vi "master_python_v1.0.vi"() -> ()   [LabVIEW 2026]
uses:
  <vilib>/Utility/error.llb/DialogType.ctl
  <vilib>/DAQmx/write.llb/DAQmx Write (Analog 2D DBL NChan NSamp).vi
  <vilib>/DAQmx/read.llb/DAQmx Read (Analog 1D Wfm NChan NSamp Duration).vi
  <vilib>/DAQmx/read.llb/DAQmx Read (Analog 1D Wfm NChan NSamp).vi
  <vilib>/DAQmx/miscellaneous.llb/DAQmx Fill In Error Info.vi
  <vilib>/Utility/inputDevices.llb/keyboardAcquire.vi
  Nanostage/Madlib.dll
panel:
  out "PID output":dbl format="%.2f"
  out "Setpoint":dbl
  in  "PID gains":T1={"proportional gain (Kc)"=0.5, "integral time (Ti, min)"=0.0, "derivative time (Td, min)"=0.0} {"derivative time (Td, min)" min=-1e-18 max=1000000000000000.0 step=1e-05 format="%.3f"; "integral time (Ti, min)" min=-1e-18 step=1e-05 format="%.6f"; "proportional gain (Kc)" min=-1e-18 step=1e-05 format="%.5f"}
  in  "output range":cluster{"output high":dbl, "output low":dbl}={"output high"=0.1, "output low"=-0.1} {"output low" format="%.2f"; "output high" format="%.2f"}
  in  "dt (s)":dbl=-1.0 format="%.3f"
  out "QPD":dbl
  out "Pos 0":dbl
  in  "Comment":string
  out "loop iteration":i32
  out "x start":dbl
  out "y start":dbl
  out "z start":dbl
  out "start iteration":dbl
  out "data":waveform(dbl)[](array[waveform])
  out "Numeric 2":i32
  out "Numeric":i32
  out "stop Ind":bool
  in  "Tab Control":enum32{"Main Control", "Calibration"}(tab)
  in  "Apply Force":bool
  out "Waveform Chart 6":waveform(dbl)(graph)
  out "Waveform Chart 5":waveform(dbl)(graph)
  in  "stop":bool
  in  "Record Data":bool
  in  "New File?":bool caption="new_file"
  out "QPD Position":cluster{"Array":dbl[], "Array":dbl[]}(graph)
  out "MT channels":waveform(dbl)[](graph)
  out "QPD Precise Position":cluster{"Array":dbl[], "Array":dbl[]}(graph)
  out "QPD Sum (Volt)":waveform(dbl)(graph)
  out "x":dbl
  out "y":dbl
  out "z":dbl
  in  "<":bool
  in  ">":bool
  in  "v":bool
  in  "^":bool
  in  "Down":bool
  in  "Up":bool
  in  "Fine":dbl=50.0
  in  "Step Size (nm)":bool
  in  "Course":dbl=500.0
  in  "Enable\ntapping":bool
  in  "DELAY (ms)":u32=10
  in  "x amplitude\n(um)":dbl
  in  "speed":i32=1
  in  "z amplitude (um)":dbl
  out "# oscillations":dbl
  in  "y amplitude\n(um)":dbl min=-25.0 max=25.0 step=0.05
  in  "Samples":u16=100 min=1 step=1
  in  "Centre":bool
  in  "Power Spectrum":bool
  in  "Duration (s)":dbl=2.0
  in  "Boolean":bool
  in  "Frequency":dbl=1.0 min=0.0 max=100.0 step=0.01
  in  "Amplitude":dbl=0.5 min=0.1 max=0.9 step=0.1
  in  "# Cycles":dbl=50.0 min=0.0 max=10000.0 step=0.001
  in  "Start Signal\nGen":bool
  in  "Desired Force (pN)":dbl step=0.01
  out "Measured Force (pN)":dbl(slide) scale=-2.0..2.0
  in  "Save Spectrum":bool
  in  "#":i32=1
  out "QPD nLR":waveform(dbl)(graph)
  out "QPD nBT":waveform(dbl)(graph)
  in  "Filename":path=path "C:/Users/localadmin/Desktop/220601 beadscan/7umscan2umbead.lvm"
  in  "Set 0 pN Position":bool
  out "QPD0":dbl
  in  "reinitialize?":bool
  in  "Conversion factor (pN/V)":dbl=1.0
  # "Left= anticlockwise"
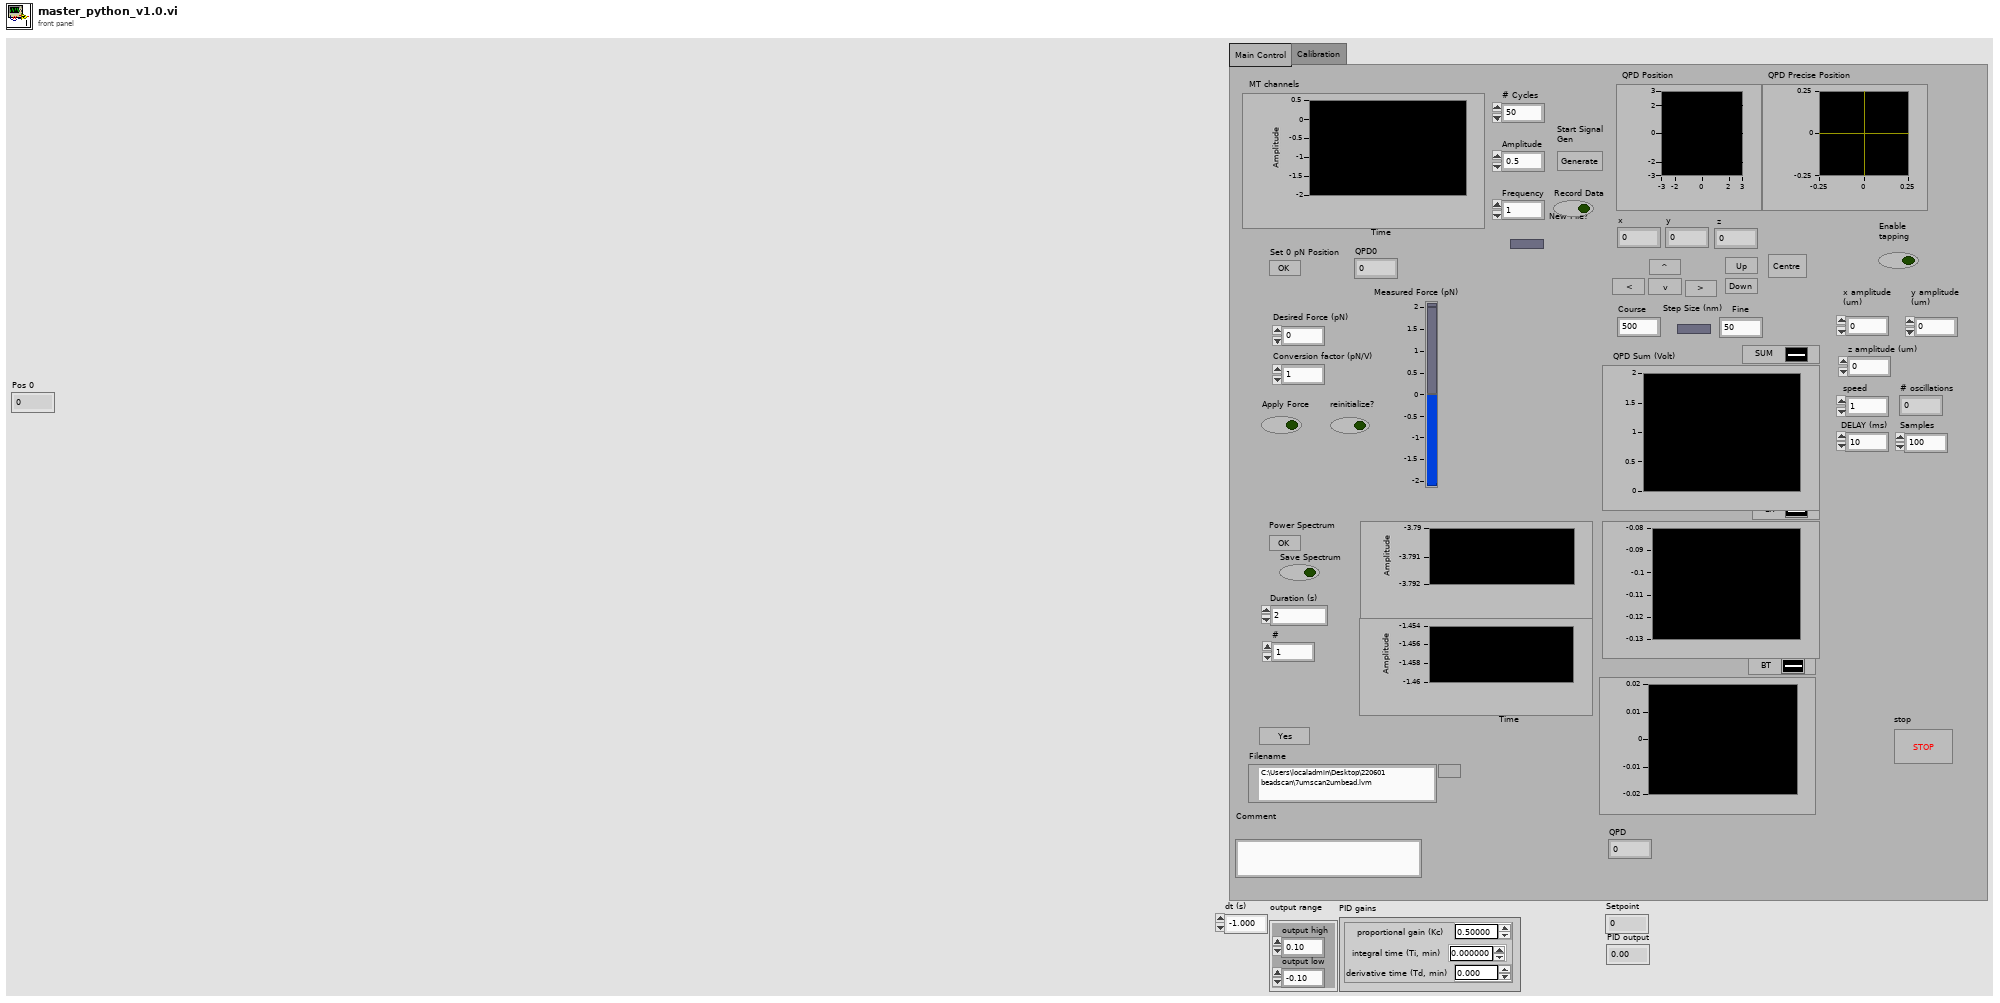
[diagram p1: front panel]
types:
  T1 = cluster{"proportional gain (Kc)":dbl, "integral time (Ti, min)":dbl, "derivative time (Td, min)":dbl}
  T2 = typedef "DialogType.ctl" = u16
  T3 = enum16{"Centre", "Move", "Tapping", "Calibration"}
  T4 = cluster{"kp":dbl, "ti":dbl, "td":dbl, "index":i32, "process_variable":dbl, "derivative_action":dbl, "integrated_error":dbl, "error":dbl, "output":dbl}
  T5 = enum16{"0", "1", "2", "3", "4", "5", "6", "7", "8", "9", "A", "B", "C", "D", "E", "F", "G", "H", "I", "J", "K", "L", "M", "N", "O", "P", "Q", "R", "S", "T", "U", "V", "W", "X", "Y", "Z", "F1", "F2", "F3", "F4", "F5", "F6", "F7", "F8", "F9", "F10", "F11", "F12", "F13", "F14", "F15", "ADD", "BACK", "BACKSLASH", "CAPITAL", "COMMA", "DECIMAL", "DELETE", "DIVIDE", "DOWN", "END", "EQUALS", "ESCAPE", "GRAVE (`)", "HOME", "INSERT", "LBRACKET", "LCONTROL", "LEFT", "L ALT", "LSHIFT", "LWIN", "MINUS", "MULTIPLY", "NEXT", "NUMLOCK", "NUMPAD_0", "NUMPAD_1", "NUMPAD_2", "NUMPAD_3", "NUMPAD_4", "NUMPAD_5", "NUMPAD_6", "NUMPAD_7", "NUMPAD_8", "NUMPAD_9", "PAUSE", "PERIOD", "PRIOR (PG UP)", "RBRACKET", "RCONTROL", "RETURN", "RIGHT", "R ALT", "RSHIFT", "RWIN", "SCROLL", "SEMICOLON", "SLASH", "SPACE", "SUBTRACT", "TAB", "UP", "ENTER (num pad)", "' (quote)"}[]
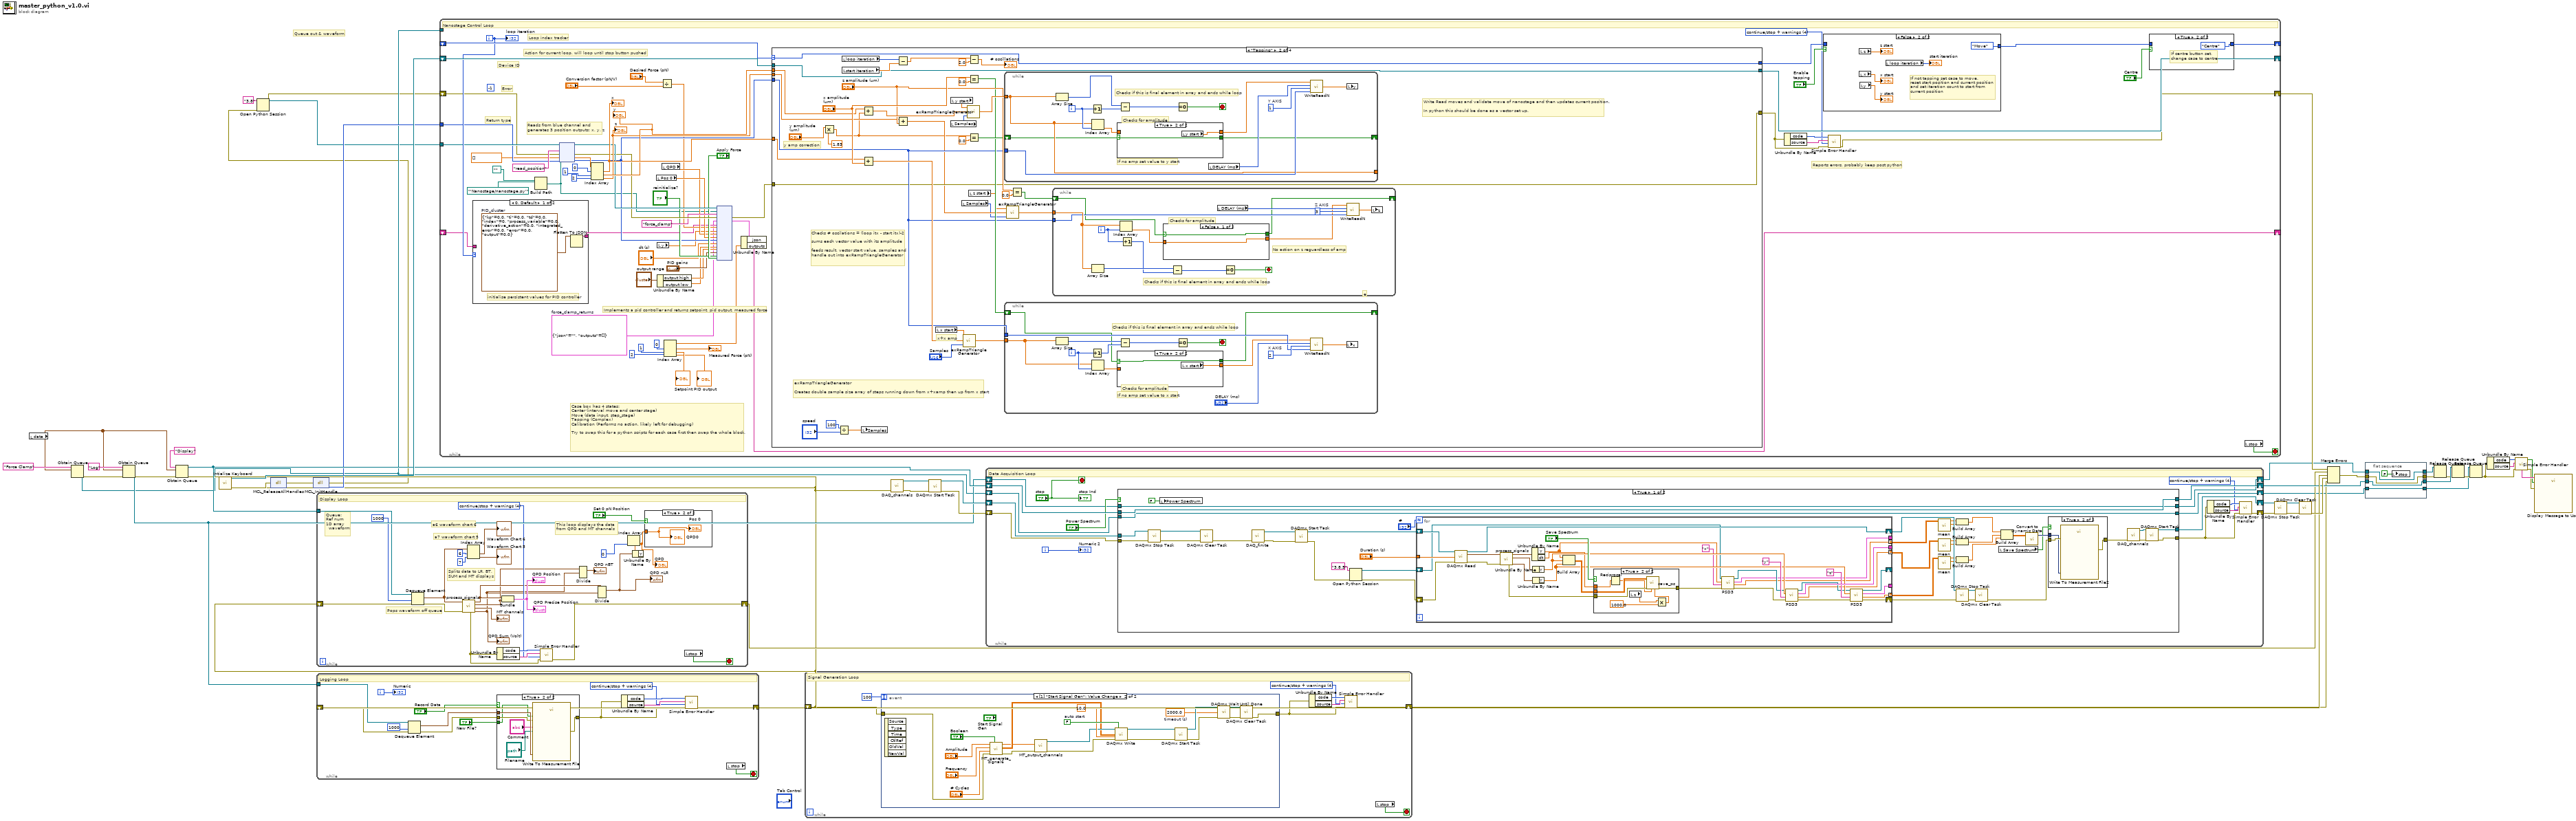
[diagram p0: block diagram]
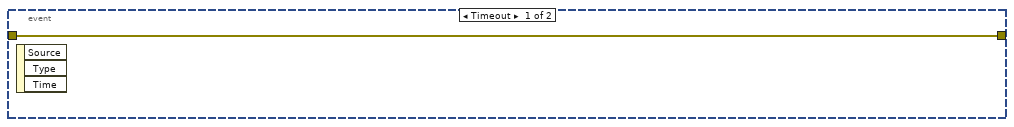
[diagram p2: hidden frame]
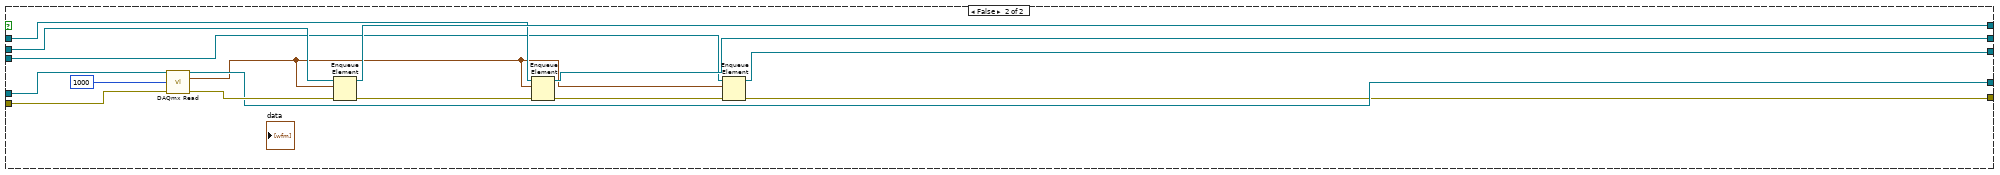
[diagram p5: hidden frame]
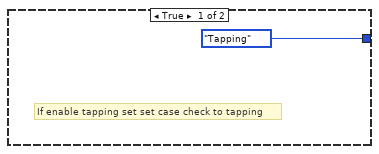
[diagram p9: hidden frame]
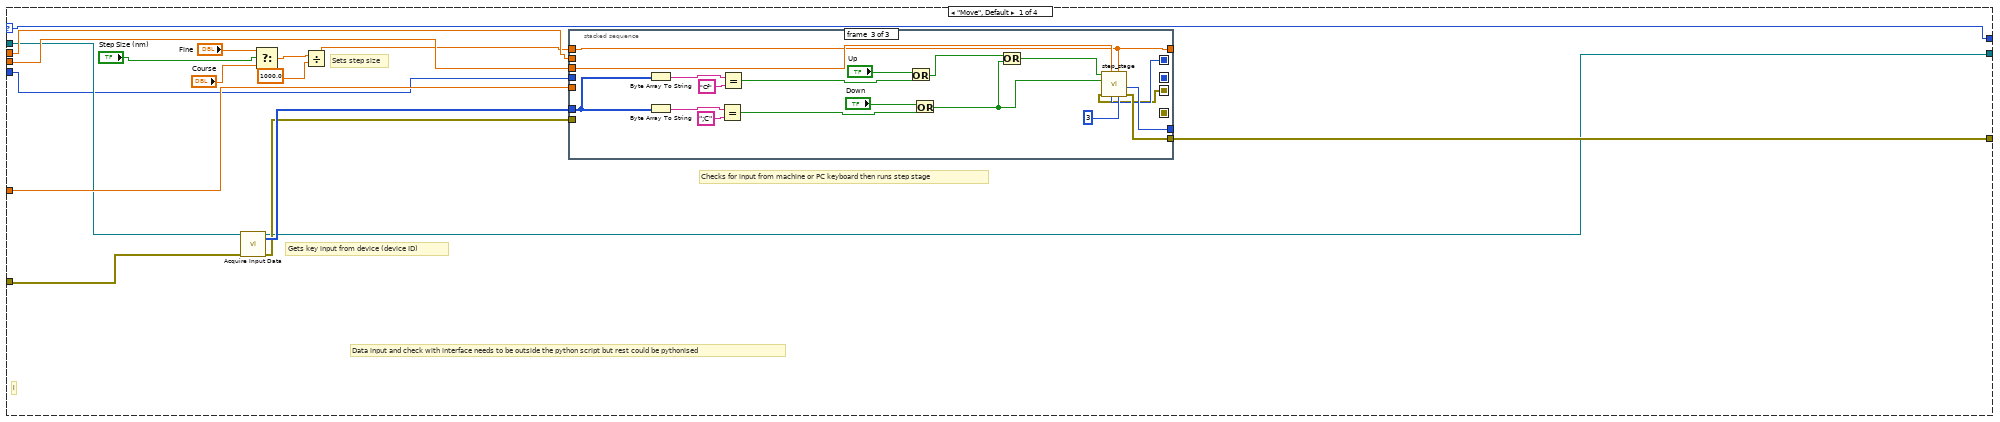
[diagram p10: hidden frame]
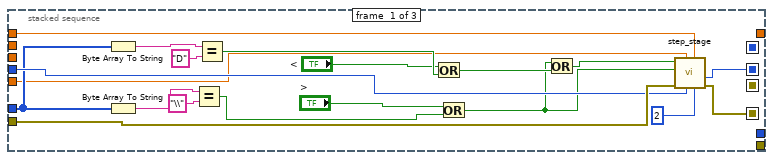
[diagram p11: hidden frame]
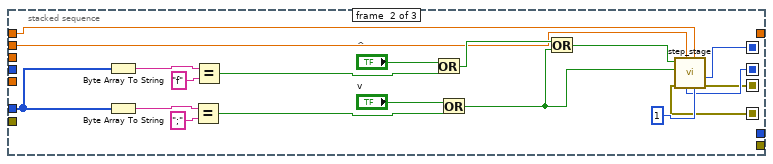
[diagram p12: hidden frame]
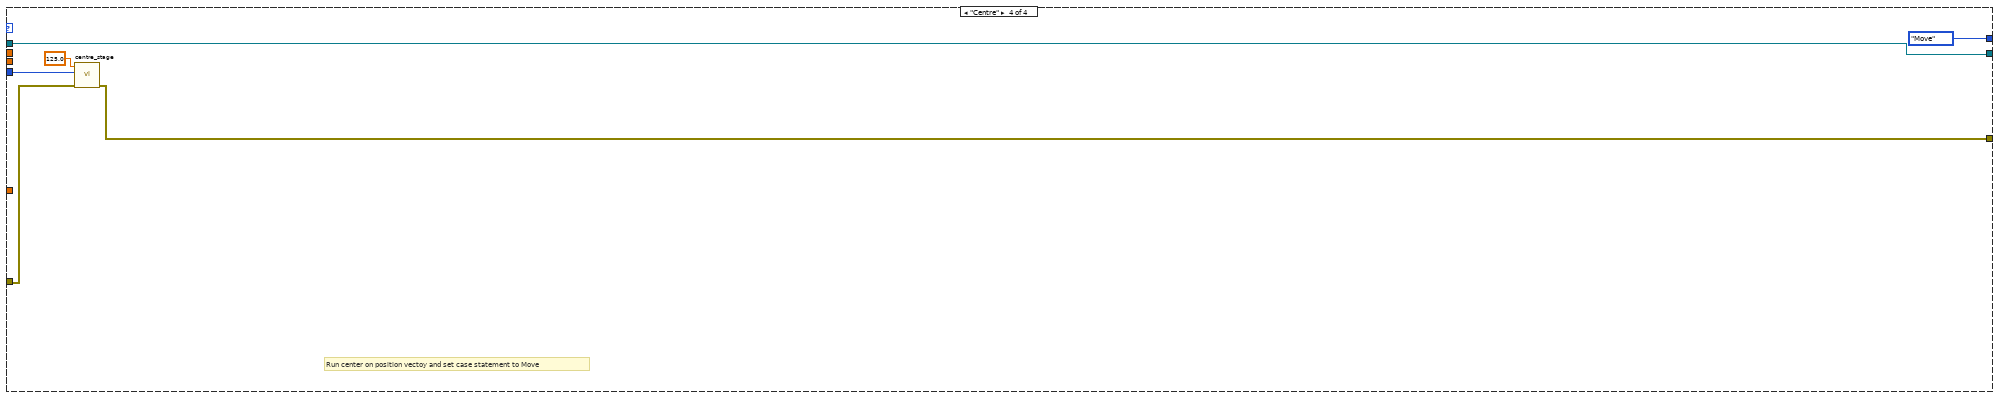
[diagram p17: hidden frame]
diagram:
  # "Queue out & waveform"
  n1 = local read "data"() -> (w10:waveform(dbl)[])
  n2 = Obtain Queue(name (unnamed)="Force Clamp", element data type=w10) -> (queue out=w5:refnum<queue>, error out=w12:errorcluster)  [unwired: 3 in, 1 out]
  n3 = Obtain Queue(name (unnamed)="Log", element data type=w10, error in (no error)=w12) -> (queue out=w16:refnum<queue>, error out=w21:errorcluster)  [unwired: 2 in, 1 out]
  n4 = Obtain Queue(name (unnamed)="Display", element data type=w10, error in (no error)=w21) -> (queue out=w23:refnum<queue>, error out=w14:errorcluster)  [unwired: 2 in, 1 out]
  n5 = call <vilib>:"Intialize Keyboard.vi"("error in (no error)"=w14) -> ("error out"=w26:errorcluster, "device ID"=w25:refnum<k1>)  [unwired: 9 out]
  n6 = dll-call lib="C:/Users/psmr500/PycharmProjects/COMBI-Tweez/LabVIEW Microscope Control/Nanostage/MADLib.dll" fn="MCL_ReleaseAllHandles"(error in=w26) -> (error out=w27:errorcluster)  [unwired: 3 in, 1 out]
  n7 = dll-call lib="C:/Users/psmr500/PycharmProjects/COMBI-Tweez/LabVIEW Microscope Control/Nanostage/MADLib.dll" fn="MCL_InitHandle"(error in=w27) -> (error out=w2:errorcluster, "return type"=w15:i32)  [unwired: 2 in, 1 out]
  n8 = Open Python Session(python version="3.8" ("Python version"), 3:w2) -> (session out=w4:refnum<k35>, error out=w3:errorcluster)  [unwired: 1 in]
  n9 = while {
    tunnel: w23 -> [w73]
    shift-right: [w58] -> w29
    shift-left: w14 -> [w72]
    stop <- w71 stop-if-true
    w57 = T2 4 items=["no dialog", "OK message", "continue or stop message", "OK message + warnings", "continue/stop + warnings"] ("type of dialog (OK msg:1)")
    # "a7 waveform chart 5"
    # "a6 waveform chart 6"
    # "Splits data to LR, BT,\nSUM and MT displays"
    # "Pops waveform off queue"
    # "Queue:\nRef num\n1D array\n  waveform"
    # "This loop displays the data from QPD and MT channels"
    # "Display Loop"
    n10 = Dequeue Element(queue=w73, timeout in ms (-1)=1000, error in (no error)=w72) -> (element=w63:waveform(dbl)[], error out=w65:errorcluster)  [unwired: 2 out]
    n11 = call "process_signals.vi"("error in (no error)"=w65, "data"=w63) -> ("SUM"=w53:waveform(dbl), "MT"=→"MT channels":waveform(dbl)[], "BT"=w54:waveform(dbl), "LR"=w55:waveform(dbl), "error out"=w66:errorcluster)  [unwired: 5 in]
    "QPD Sum (Volt)" <- w53
    n12 = Index Array(array=w63, index #1=6 ("index"), index #2=7 ("index")) -> (element #1=→"Waveform Chart 6":waveform(dbl), element #2=→"Waveform Chart 5":waveform(dbl))
    n13 = Unbundle By Name(w66) -> ("code"=w68:i32, "source"=w67:string)
    n14 = Bundle("LR"=w55, "BT"=w54) -> (→"QPD Position" →"QPD Precise Position":cluster{"LR":waveform(dbl), "BT":waveform(dbl)})  [unwired: 1 in]
    n15 = call <vilib>:"Simple Error Handler.vi"("error code (no error:0)"=w68, "error source (\" \")"=w67, "type of dialog (OK msg:1)"=w57, "error in (no error)"=w66) -> ("error out"=w58:errorcluster)  [unwired: 1 in, 4 out]
    n16 = Divide(1:w53, 2:w54) -> (0:→"QPD nBT":waveform(dbl))  [unwired: 1 in, 1 out]
    n17 = Divide(1:w53, 2:w55) -> (0:w50:waveform(dbl))  [unwired: 1 in, 1 out]
    "QPD nLR" <- w50
    n18 = Unbundle By Name(w50) -> ("Y"=w51:dbl[])
    n19 = Index Array(array=w51, index=0) -> (element=w48:dbl)
    "QPD" <- w48
    n20 = case shown="True" "Set 0 pN Position" {
      tunnel: w48 -> [_ w74]
      frame False {
      }
      frame True {
        "Pos 0" <- w74
        "QPD0" <- w74
      }
    }
    n21 = local read "stop"() -> (w71:bool)
  }
  n22 = while {
    shift-right: [w76] -> w33
    shift-left: w14 -> [w88]
    tunnel: w16 -> [w87]
    i -> [w82]
    stop <- w77 stop-if-true
    w75 = T2 4 items=["no dialog", "OK message", "continue or stop message", "OK message + warnings", "continue/stop + warnings"] ("type of dialog (OK msg:1)")
    # "Logging Loop"
    n23 = Dequeue Element(queue=w87, timeout in ms (-1)=1000, error in (no error)=w88) -> (element=w84:waveform(dbl)[], error out=w85:errorcluster)  [unwired: 2 out]
    n24 = case shown="True" "Record Data" {
      tunnel: [w89 w95] -> w78
      tunnel: w84 -> [_ w94]
      tunnel: "New File?" -> [_ w91]
      tunnel: w85 -> [w89 w93]
      frame False {
      }
      frame True {
        n25 = call "Write To Measurement File"("Signals"=w94, "new_file"=w91, "error in (no error)"=w93, "Filename"="Filename", "Comment"="Comment") -> ("error out"=w95:errorcluster)  [unwired: 12 in, 2 out]
      }
    }
    n26 = Unbundle By Name(w78) -> ("code"=w80:i32, "source"=w79:string)
    n27 = call <vilib>:"Simple Error Handler.vi"("error code (no error:0)"=w80, "error source (\" \")"=w79, "type of dialog (OK msg:1)"=w75, "error in (no error)"=w78) -> ("error out"=w76:errorcluster)  [unwired: 1 in, 4 out]
    n28 = local read "stop"() -> (w77:bool)
    "Numeric" <- w82
  }
  n29 = while {
    shift-right: [w144] -> w24
    shift-left: w3 -> [w135]
    shift-right: [w149] -> _
    shift-left: w25 -> [w151]
    shift-right: [w145] -> _
    shift-left: _ -> [w150]
    tunnel: w15 -> [w134]
    tunnel: w5 -> [_]
    shift-right: [w106] -> _
    shift-left: _ -> [w138]
    tunnel: w4 -> [w136]
    i -> [w139]
    stop <- w155 stop-if-true
    w108 = cluster{"json":string, "outputs":dbl[]} {"json"="", "outputs"=[]}  # force_clamp_returns
    (unwired) -1 ("timeout in ms (-1)")
    w143 = T2 4 items=["no dialog", "OK message", "continue or stop message", "OK message + warnings", "continue/stop + warnings"] ("type of dialog (OK msg:1)")
    # "Reports errors, probably keep post python"
    # "Case box has 4 states:\nCenter (interval move and center stage)\nMove (data input, step_stage)\nTapping (Complex)\nCalibration (Performs no action, likely left for debugging)\n\nTry to swap this for a python scripts for each case first then swap the whole block."
    # "Action for current loop, will loop until stop button pushed"
    # "Implements a pid controller and returns setpoint, pid output, measured force"
    # "Return type"
    # "Device ID"
    # "Error"
    # "Reads from blue channel and \ngenerates 3 position outputs: x, y, z"
    # "Loop index tracker"
    # "Nanostage Control Loop"
    n30 = case shown="0, Default" w139 {
      tunnel: [w156 w158] -> w109
      tunnel: w138 -> [_ w158]
      frame 0, Default {
        w157 = T4 {"kp"=0.0, "ti"=0.0, "td"=0.0, "index"=0, "process_variable"=0.0, "derivative_action"=0.0, "integrated_error"=0.0, "error"=0.0, "output"=0.0}  # PID_cluster
        # "initialise persistent values for PID controller"
        n31 = Flatten To JSON(anything=w157) -> (JSON string=w156:string)  [unwired: 2 in, 1 out]
      }
      frame 1 {
      }
    }
    n32 = Build Path(base path=path "", name or relative path=path "'Nanostage/nanostage.py'") -> (appended path=w96:path)
    n33 = node(w136, w96, "read_position" ("function name"), w135, dbl[] [], w134) -> (w125:refnum<k35>, w124:errorcluster, w132:dbl[], w114:i32)  [unwired: 2 out]
    n34 = Index Array(array=w132, index #1=0 ("index"), index #2=1 ("index"), index #3=2 ("index")) -> (element #1=w128:dbl, element #2=w127:dbl, element #3=w126:dbl)
    "x" <- w128
    "y" <- w127
    "z" <- w126
    n35 = local read "Pos 0"() -> (w113:dbl)
    n36 = Unbundle By Name("output range") -> ("output high"=w117:dbl, "output low"=w116:dbl)
    n37 = local read "y"() -> (w111:dbl)
    n38 = Divide(x="Desired Force (pN)", y="Conversion factor (pN/V)") -> (x/y=w110:dbl)
    n39 = local read "QPD"() -> (w112:dbl)
    n40 = node(w125, w96, "force_clamp" ("function name"), w124, w108, w109, w110, w111, w112, w113, w114, "dt (s)", w116, w117, "PID gains", "reinitialize?", "Apply Force") -> (w123:errorcluster, w107:cluster{"json":string, "outputs":dbl[]})  [unwired: 12 in, 3 out]
    n41 = Unbundle By Name(w107) -> ("json"=w106:string, "outputs"=w105:dbl[])
    n42 = Index Array(array=w105, index #1=0 ("index"), index #2=1 ("index"), index #3=2 ("index")) -> (element #1=→"Measured Force (pN)":dbl, element #2=→"Setpoint":dbl, element #3=→"PID output":dbl)
    n43 = case shown="\"Tapping\"" w150 {
      selector: w150 -> [w167 w251 w342 _]
      tunnel: w123 -> [w173 w253 w340 w357]
      tunnel: w114 -> [w171 w254 w341 w356]
      tunnel: [w169 w253 w334 w355] -> w152
      tunnel: w128 -> [w183 w256 w344 _]
      tunnel: w127 -> [w182 w255 w343 _]
      tunnel: w126 -> [w181 w250 _ _]
      tunnel: w151 -> [w174 w252 w333 w352]
      tunnel: [w167 w251 w342 T3."Move"] -> w148
      tunnel: [w168 w252 w333 w352] -> w149
      frame "Move", Default {
        # "Data input and check with interface needs to be outside the python script but rest could be pythonised"
        # "Checks for input from machine or PC keyboard then runs step stage"
        # "Sets step size"
        # "Gets key input from device (device ID)"
        # "l"
        n44 = call-poly <vilib>:"Acquire Input Data.vi"("device ID"=w174, "error in (no error)"=w173) -> ("device ID"=w168:refnum<k1>, "keys pressed"=w172:T5, "error out"=w170:errorcluster)  [unwired: 15 out]
        n45 = Select(t="Fine", s="Step Size (nm)", f="Course") -> (s? t:f=w177:dbl)
        n46 = Divide(x=w177, y=1000.0) -> (x/y=w175:dbl)
        n47 = stacked-sequence {
          seq-local: [w199 _ _] -> [_ w220 _]
          seq-local: [w198 _ _] -> [_ w219 _]
          seq-local: [_ w217 _] -> [_ _ w236]
          seq-local: [_ w218 _] -> [_ _ w235]
          tunnel: w170 -> [w202 _ _]
          tunnel: w171 -> [w201 _ _]
          tunnel: w183 -> [w185 _ _]
          tunnel: w182 -> [_ w204 _]
          tunnel: w181 -> [_ _ w239]
          tunnel: [_ _ w237] -> w169
          tunnel: [_ _ w238] -> _
          tunnel: w172 -> [w187 w206 w223]
          tunnel: [_ _ w222] -> _
          tunnel: w175 -> [w186 w205 w222]
          frame #0 {
            n48 = Byte Array To String(unsigned byte array=w187) -> (string=w195:string)
            n49 = Byte Array To String(unsigned byte array=w187) -> (string=w197:string)
            n50 = Equal?(x=w197, y="\\") -> (x = y?=w193:bool)
            n51 = Equal?(x=w195, y="D") -> (x = y?=w192:bool)
            n52 = Or(x="<", y=w192) -> (x .or. y?=w189:bool)
            n53 = Or(x=">", y=w193) -> (x .or. y?=w184:bool)
            n54 = Or(x=w184, y=w189) -> (x .or. y?=w188:bool)
            n55 = call "step_stage.vi"("axis"=u32 2, "step"=w186, "handle"=w201, "position"=w185, "error in"=w202, "+/-"=w184, "move"=w188) -> ("error out"=w198:errorcluster, "handle out"=w199:i32)  [unwired: 3 in]
          }
          frame #1 {
            n56 = Byte Array To String(unsigned byte array=w206) -> (string=w216:string)
            n57 = Byte Array To String(unsigned byte array=w206) -> (string=w214:string)
            n58 = Equal?(x=w214, y=";") -> (x = y?=w209:bool)
            n59 = Equal?(x=w216, y="f") -> (x = y?=w212:bool)
            n60 = Or(x="^", y=w212) -> (x .or. y?=w208:bool)
            n61 = Or(x="v", y=w209) -> (x .or. y?=w207:bool)
            n62 = Or(x=w208, y=w207) -> (x .or. y?=w203:bool)
            n63 = call "step_stage.vi"("axis"=u32 1, "step"=w205, "handle"=w220, "position"=w204, "error in"=w219, "+/-"=w207, "move"=w203) -> ("error out"=w218:errorcluster, "handle out"=w217:i32)  [unwired: 3 in]
          }
          frame #2 {
            n64 = Byte Array To String(unsigned byte array=w223) -> (string=w234:string)
            n65 = Byte Array To String(unsigned byte array=w223) -> (string=w232:string)
            n66 = Equal?(x=w232, y=";C") -> (x = y?=w229:bool)
            n67 = Equal?(x=w234, y="Cf") -> (x = y?=w230:bool)
            n68 = Or(x="Up", y=w230) -> (x .or. y?=w228:bool)
            n69 = Or(x="Down", y=w229) -> (x .or. y?=w226:bool)
            n70 = Or(x=w228, y=w226) -> (x .or. y?=w227:bool)
            n71 = call "step_stage.vi"("axis"=u32 3, "step"=w222, "handle"=w236, "position"=w239, "error in"=w235, "+/-"=w226, "move"=w227) -> ("error out"=w237:errorcluster, "handle out"=w238:i32)  [unwired: 3 in]
          }
        }
      }
      frame "Tapping" {
        # "Write Read moves and validate move of nanostage and then updates current position.\n\nIn python this should be done as a vector set up."
        # "exRampTriangleGenerator\n\nCreates double sample size array of steps running down from x+xamp then up from x start"
        # "Checks # oscilations = (loop itx - start itx)-2\n\nsums each vector value with its amplitude\n\nfeeds result, vector start value, samples and \nhandle out into exRampTriangleGenerator"
        # "x+x amp"
        # "y amp correction"
        n72 = Multiply(x="y amplitude\n(um)", y=1.83) -> (x*y=w242:dbl)
        n73 = Divide(x=100, y="speed") -> (x/y=w273:dbl)
        n74 = local read "loop iteration"() -> (w268:i32)
        n75 = local read "start iteration"() -> (w269:dbl)
        n76 = local write "Samples"(w273) -> ()
        n77 = Add(x=w255, y=w242) -> (x+y=w272:dbl)
        n78 = Add(x=w256, y="x amplitude\n(um)") -> (x+y=w277:dbl)
        n79 = Subtract(x=w268, y=w269) -> (x-y=w267:dbl)
        n80 = Add(x=w250, y="z amplitude (um)") -> (x+y=w249:dbl)
        n81 = local read "x start"() -> (w246:dbl)
        n82 = local read "Samples"() -> (w270:u16)
        n83 = local read "y start"() -> (w244:dbl)
        n84 = local read "Samples"() -> (w248:u16)
        n85 = call "exRampTriangleGenerator.vi"("Number of positions"="Samples", "End(um)"=w277, "Start(um)"=w246) -> ("Array"=w278:dbl[])
        n86 = call "exRampTriangleGenerator.vi"("Number of positions"=w270, "End(um)"=w272, "Start(um)"=w244) -> ("Array"=w271:dbl[])
        n87 = Subtract(x=w267, y=2.0) -> (x-y=→"# oscillations":dbl)
        n88 = Equal?(x="x amplitude\n(um)", y=0.0) -> (x = y?=w258:bool)
        n89 = Equal?(x=w242, y=0.0) -> (x = y?=w259:bool)
        n90 = local read "z start"() -> (w245:dbl)
        n91 = while {
          tunnel: [w302] -> _
          tunnel: w254 -> [w309]
          tunnel: w271 -> [w302]
          shift-right: [w298] -> _
          shift-left: w259 -> [w299]
          i -> [w310]
          stop <- w304 stop-if-true
          w305 = 1  # Y AXIS
          # "If no amp set value to y start"
          # "Checks if this is final element in array and ends while loop"
          # "Checks for amplitude"
          n92 = Array Size(array=w302) -> (size(s)=w307:i32)
          n93 = Increment(x=w310) -> (x+1=w306:i32)
          n94 = Index Array(array=w302, index=w310) -> (element=w301:dbl)
          n95 = case shown="True" w299 {
            selector: w299 -> [w311 w314]
            tunnel: w301 -> [w312 _]
            tunnel: [w312 w313] -> w300
            tunnel: [w311 w314] -> w298
            frame False {
            }
            frame True {
              n96 = local read "y start"() -> (w313:dbl)
            }
          }
          n97 = Subtract(x=w307, y=w306) -> (x-y=w308:i32)
          n98 = Equal To 0?(x=w308) -> (x = 0?=w304:bool)
          n99 = local read "DELAY (ms)"() -> (w303:u32)
          n100 = call "WriteReadN.vi"("Handle"=w309, "Axis"=w305, "Delay (ms)"=w303, "Move to (um)"=w300) -> ("Current Position (um)"=w297:dbl)
          n101 = local write "y"(w297) -> ()
        }
        n102 = while {
          tunnel: w278 -> [w320]
          tunnel: w254 -> [w321]
          shift-right: [w316] -> _
          shift-left: w258 -> [w317]
          i -> [w324]
          stop <- w326 stop-if-true
          w322 = 2  # X AXIS
          # "If no amp set value to x start"
          # "Checks if this is final element in array and ends while loop"
          # "Checks for amplitude"
          n103 = Array Size(array=w320) -> (size(s)=w327:i32)
          n104 = Increment(x=w324) -> (x+1=w325:i32)
          n105 = Index Array(array=w320, index=w324) -> (element=w319:dbl)
          n106 = case shown="True" w317 {
            selector: w317 -> [w329 w332]
            tunnel: w319 -> [w330 _]
            tunnel: [w330 w331] -> w318
            tunnel: [w329 w332] -> w316
            frame False {
            }
            frame True {
              n107 = local read "x start"() -> (w331:dbl)
            }
          }
          n108 = Subtract(x=w327, y=w325) -> (x-y=w328:i32)
          n109 = Equal To 0?(x=w328) -> (x = 0?=w326:bool)
          n110 = call "WriteReadN.vi"("Handle"=w321, "Axis"=w322, "Delay (ms)"="DELAY (ms)", "Move to (um)"=w318) -> ("Current Position (um)"=w315:dbl)
          n111 = local write "x"(w315) -> ()
        }
        n112 = call "exRampTriangleGenerator.vi"("Number of positions"=w248, "End(um)"=w249, "Start(um)"=w245) -> ("Array"=w247:dbl[])
        n113 = Equal?(x="z amplitude (um)", y=0.0) -> (x = y?=w257:bool)
        n114 = while {
          tunnel: w247 -> [w285]
          tunnel: w254 -> [w284]
          shift-right: [w280] -> _
          shift-left: w257 -> [w281]
          i -> [w288]
          stop <- w290 stop-if-true
          w287 = 3  # Z AXIS
          # "No action on z reguardless of amp"
          # "Checks if this is final element in array and ends while loop"
          # "Checks for amplitude"
          # "e"
          n115 = Array Size(array=w285) -> (size(s)=w291:i32)
          n116 = Index Array(array=w285, index=w288) -> (element=w283:dbl)
          n117 = Increment(x=w288) -> (x+1=w289:i32)
          n118 = case shown="False" w281 {
            selector: w281 -> [w293 w296]
            tunnel: w283 -> [w294 w295]
            tunnel: [w294 w295] -> w282
            tunnel: [w293 w296] -> w280
            frame False {
            }
            frame True {
            }
          }
          n119 = Subtract(x=w291, y=w289) -> (x-y=w292:i32)
          n120 = local read "DELAY (ms)"() -> (w286:u32)
          n121 = Equal To 0?(x=w292) -> (x = 0?=w290:bool)
          n122 = call "WriteReadN.vi"("Handle"=w284, "Axis"=w287, "Delay (ms)"=w286, "Move to (um)"=w282) -> ("Current Position (um)"=w279:dbl)
          n123 = local write "z"(w279) -> ()
        }
      }
      frame "Calibration" {
        n124 = flat-sequence {
          tunnel: w340 -> [w345]
          tunnel: [w345] -> w335
          tunnel: [w346] -> w336
          tunnel: w335 -> [w346]
          tunnel: w341 -> [_]
          tunnel: w344 -> [_]
          tunnel: w343 -> [_]
          tunnel: [w347] -> w337
          tunnel: w336 -> [w347]
          tunnel: [w348] -> w338
          tunnel: w337 -> [w348]
          tunnel: [w350] -> _
          tunnel: w341 -> [w350]
          tunnel: [w349] -> w339
          tunnel: w338 -> [w349]
          tunnel: w339 -> [w351]
          tunnel: [w351] -> w334
          frame #0 {
          }
          frame #1 {
          }
          frame #2 {
          }
          frame #3 {
          }
          frame #4 {
          }
          frame #5 {
          }
        }
      }
      frame "Centre" {
        # "Run center on position vectoy and set case statement to Move"
        n125 = call "centre_stage.vi"("error in"=w357, "handle in"=w356, "Destination"=125.0) -> ("error out"=w355:errorcluster)  [unwired: 7 in, 1 out]
      }
    }
    n126 = Unbundle By Name(w152) -> ("code"=w154:i32, "source"=w153:string)
    n127 = case shown="False" "Enable\ntapping" {
      tunnel: w148 -> [_ _]
      tunnel: [T3."Tapping" T3."Move"] -> w142
      frame True {
        # "If enable tapping set set case check to tapping"
      }
      frame False {
        # "If not tapping set case to move.\nreset start position and current position \nand set iteration count to start from \ncurrent position"
        n128 = local read "z"() -> (→"z start":dbl)
        n129 = local read "x"() -> (→"x start":dbl)
        n130 = local read "y"() -> (→"y start":dbl)
        n131 = local read "loop iteration"() -> (→"start iteration":i32)
      }
    }
    n132 = call <vilib>:"Simple Error Handler.vi"("error code (no error:0)"=w154, "error source (\" \")"=w153, "type of dialog (OK msg:1)"=w143, "error in (no error)"=w152) -> ("error out"=w144:errorcluster)  [unwired: 1 in, 4 out]
    n133 = case shown="True" "Centre" {
      tunnel: [w159 T3."Centre"] -> w145
      tunnel: w142 -> [w159 _]
      frame False {
        # "If not centre no effect"
      }
      frame True {
        # "If centre button set, \nchange case to centre"
      }
    }
    n134 = local read "stop"() -> (w155:bool)
    "loop iteration" <- w139
  }
  n135 = while {
    shift-right: [w359] -> w13
    shift-left: w14 -> [w364]
    stop <- w365 stop-if-true
    w360 = T2 4 items=["no dialog", "OK message", "continue or stop message", "OK message + warnings", "continue/stop + warnings"] ("type of dialog (OK msg:1)")
    # "Signal Generation Loop"
    n136 = event shown="[1] \"Start Signal Gen\": Value Change" {
      selector: _ -> [_ _]
      dyn-events: _ -> [_ _]
      timeout: 100 -> [_ _]
      tunnel: [w366 w369] -> w358
      tunnel: w364 -> [w366 w368]
      event Timeout {
        n137 = event-data() -> ()  [unwired: 1 in, 3 out]
      }
      event "Start Signal\nGen": Value Change {
        w378 = 2000.0  # timeout (s)
        w377 = FALSE  # auto start
        n138 = event-data() -> ()  [unwired: 1 in, 6 out]
        n139 = call "MT_generate_signal6.vi"("Direction"="Boolean", "error in (no error)"=w368, "# cycles"="# Cycles", "frequency"="Frequency", "amplitude"="Amplitude") -> ("error out"=w374:errorcluster, "signals out"=w372:dbl[][], "# samples"=w371:dbl)  [unwired: 4 in]
        n140 = call "MT_output_channels.vi"("error in"=w374, "number of samples"=w371) -> ("error out"=w373:errorcluster, "task out"=w375:refnum<k21>)  [unwired: 8 in]
        n141 = call-poly <vilib>:"DAQmx Write.vi"("task/channels in"=w375, "auto start"=w377, "data"=w372, "timeout"=10.0, "error in"=w373) -> ("task out"=w382:refnum<k21>, "error out"=w383:errorcluster)  [unwired: 8 in, 1 out]
        n142 = call <vilib>:"DAQmx Start Task.vi"("task/channels in"=w382, "error in"=w383) -> ("task out"=w379:refnum<k21>, "error out"=w380:errorcluster)  [unwired: 12 in]
        n143 = call <vilib>:"DAQmx Wait Until Done.vi"("task/channels in"=w379, "timeout (sec)"=w378, "error in"=w380) -> ("task out"=w384:refnum<k21>, "error out"=w381:errorcluster)  [unwired: 11 in]
        n144 = call <vilib>:"DAQmx Clear Task.vi"("task in"=w384, "error in"=w381) -> ("error out"=w369:errorcluster)  [unwired: 13 in]
      }
    }
    n145 = Unbundle By Name(w358) -> ("code"=w362:i32, "source"=w361:string)
    n146 = call <vilib>:"Simple Error Handler.vi"("error code (no error:0)"=w362, "error source (\" \")"=w361, "type of dialog (OK msg:1)"=w360, "error in (no error)"=w358) -> ("error out"=w359:errorcluster)  [unwired: 1 in, 4 out]
    n147 = local read "stop"() -> (w365:bool)
  }
  n148 = call "DAQ_channels.vi"("error in"=w14) -> ("error out"=w41:errorcluster, "task out"=w42:refnum<k21>)  [unwired: 9 in]
  n149 = call <vilib>:"DAQmx Start Task.vi"("task/channels in"=w42, "error in"=w41) -> ("task out"=w45:refnum<k21>, "error out"=w46:errorcluster)  [unwired: 12 in]
  n150 = while {
    shift-right: [w388] -> w40
    shift-left: w46 -> [w403]
    shift-right: [w400] -> w32
    shift-left: w23 -> [w401]
    shift-right: [w397] -> w28
    shift-left: w45 -> [w402]
    shift-right: [w392] -> w20
    shift-left: w16 -> [w391]
    shift-right: [w389] -> w6
    shift-left: w5 -> [w390]
    i -> [w398]
    stop <- "stop" stop-if-true
    w387 = T2 4 items=["no dialog", "OK message", "continue or stop message", "OK message + warnings", "continue/stop + warnings"] ("type of dialog (OK msg:1)")
    # "Data Acquisition Loop"
    n151 = case shown="True" "Power Spectrum" {
      tunnel: w403 -> [w445 w507]
      tunnel: w402 -> [w446 w505]
      tunnel: w401 -> [w444 w504]
      tunnel: [w444 w503] -> w400
      tunnel: [w431 w502] -> w397
      tunnel: [w430 w496] -> w393
      tunnel: w391 -> [w443 w500]
      tunnel: [w443 w498] -> w392
      tunnel: w390 -> [w428 w495]
      tunnel: [w428 w494] -> w389
      frame True {
        n152 = call <vilib>:"DAQmx Stop Task.vi"("task/channels in"=w446, "error in"=w445) -> ("task out"=w442:refnum<k21>, "error out"=w441:errorcluster)  [unwired: 12 in]
        n153 = local write "Power Spectrum"(FALSE ("Power Spectrum")) -> ()
        n154 = call <vilib>:"DAQmx Clear Task.vi"("task in"=w442, "error in"=w441) -> ("error out"=w427:errorcluster)  [unwired: 13 in]
        n155 = call "DAQ_finite.vi"("error in"=w427) -> ("error out"=w439:errorcluster, "task out"=w440:refnum<k21>)  [unwired: 9 in]
        n156 = call <vilib>:"DAQmx Start Task.vi"("task/channels in"=w440, "error in"=w439) -> ("task out"=w438:refnum<k21>, "error out"=w426:errorcluster)  [unwired: 12 in]
        n157 = Open Python Session(python version="3.8.5" ("Python version"), 3:w426) -> (session out=w423:refnum<k35>, error out=w425:errorcluster)  [unwired: 1 in]
        n158 = for {
          N: "#" -> [_]
          tunnel: "Duration (s)" -> [w481]
          tunnel: [w479] -> _
          tunnel: [w465] -> _
          tunnel: [w456] -> _
          shift-right: [w482] -> w434
          shift-left: w438 -> [w483]
          shift-right: [w463] -> _
          shift-left: w423 -> [w461]
          shift-right: [w467] -> w404
          shift-left: w425 -> [w455]
          tunnel: [w453] -> w422 mode=indexing
          tunnel: [w452] -> w421 mode=indexing
          tunnel: [w451] -> w420 mode=indexing
          n159 = call-poly <vilib>:"DAQmx Read.vi"("task/channels in"=w483, "duration"=w481, "error in"=w455) -> ("task out"=w482:refnum<k21>, "data"=w480:waveform(dbl)[], "error out"=w454:errorcluster)  [unwired: 10 in]
          n160 = call "process_signals.vi"("error in (no error)"=w454, "data"=w480) -> ("SUM"=w475:waveform(dbl), "BT"=w477:waveform(dbl), "LR"=w476:waveform(dbl), "error out"=w471:errorcluster)  [unwired: 5 in, 1 out]
          n161 = Unbundle By Name(w476) -> ("Y"=w457:dbl[], "dt"=w472:dbl)
          n162 = Unbundle By Name(w477) -> ("Y"=w474:dbl[])
          n163 = Unbundle By Name(w475) -> ("Y"=w466:dbl[])
          n164 = Build Array(w457, w474, w466) -> (w473:dbl[][])
          n165 = case shown="True" "Save Spectrum" {
            tunnel: w473 -> [_ w492]
            tunnel: w472 -> [_ w489]
            tunnel: w471 -> [w484 w491]
            tunnel: [w484 w490] -> w459
            frame False {
            }
            frame True {
              n166 = Reciprocal(x=w489) -> (1/x=w488:dbl)
              n167 = local read "z"() -> (w487:dbl)
              n168 = Multiply(x=w487, y=1000.0) -> (x*y=w486:dbl)
              n169 = call "save_ps.vi"("Height"=w486, "Rate"=w488, "error in"=w491, "QPD Data"=w492) -> ("error out"=w490:errorcluster)  [unwired: 7 in]
            }
          }
          n170 = call "PSD3.vi"("error in (no error)"=w459, "axis"="x", "data"=w457, "Refnum in"=w461) -> ("error out"=w458:errorcluster, "parameters"=w453:dbl[], "Array"=w456:cluster{dbl, dbl, dbl[]}[], "Refnum out"=w460:refnum<k35>)  [unwired: 4 in]
          n171 = call "PSD3.vi"("error in (no error)"=w458, "axis"="y", "data"=w474, "Refnum in"=w460) -> ("error out"=w468:errorcluster, "parameters"=w452:dbl[], "Array"=w479:cluster{dbl, dbl, dbl[]}[], "Refnum out"=w464:refnum<k35>)  [unwired: 4 in]
          n172 = call "PSD3.vi"("error in (no error)"=w468, "axis"="z", "data"=w466, "Refnum in"=w464) -> ("error out"=w467:errorcluster, "parameters"=w451:dbl[], "Array"=w465:cluster{dbl, dbl, dbl[]}[], "Refnum out"=w463:refnum<k35>)  [unwired: 4 in]
        }
        n173 = call "mean.vi"("parameters"=w422) -> ("k"=w415:dbl, "b"=w416:dbl)  [unwired: 9 in]
        n174 = call "mean.vi"("parameters"=w421) -> ("k"=w413:dbl, "b"=w414:dbl)  [unwired: 9 in]
        n175 = call "mean.vi"("parameters"=w420) -> ("k"=w411:dbl, "b"=w412:dbl)  [unwired: 9 in]
        n176 = Build Array(w416, w415) -> (w418:dbl[])
        n177 = Build Array(w414, w413) -> (w405:dbl[])
        n178 = Build Array(w412, w411) -> (w417:dbl[])
        n179 = call <vilib>:"DAQmx Stop Task.vi"("task/channels in"=w434, "error in"=w404) -> ("task out"=w436:refnum<k21>, "error out"=w435:errorcluster)  [unwired: 12 in]
        n180 = call <vilib>:"DAQmx Clear Task.vi"("task in"=w436, "error in"=w435) -> ("error out"=w410:errorcluster)  [unwired: 13 in]
        n181 = local read "Save Spectrum"() -> (w406:bool)
        n182 = Build Array(w418, w405, w417) -> (w408:dbl[][])
        n183 = call "Convert to Dynamic Data"("2D Array"=w408) -> ("Dynamic Data Type"=w407:dynamicdata)  [unwired: 3 in]
        n184 = case shown="True" w406 {
          tunnel: w410 -> [w447 w450]
          tunnel: [w447 w449] -> w409
          tunnel: w407 -> [_ w448]
          frame False {
          }
          frame True {
            n185 = call "Write To Measurement File2"("Signals"=w448, "error in (no error)"=w450) -> ("error out"=w449:errorcluster)  [unwired: 15 in, 2 out]
          }
        }
        n186 = call "DAQ_channels.vi"("error in"=w409) -> ("error out"=w432:errorcluster, "task out"=w433:refnum<k21>)  [unwired: 9 in]
        n187 = call <vilib>:"DAQmx Start Task.vi"("task/channels in"=w433, "error in"=w432) -> ("task out"=w431:refnum<k21>, "error out"=w430:errorcluster)  [unwired: 12 in]
      }
      frame False {
        n188 = call-poly <vilib>:"DAQmx Read.vi"("task/channels in"=w505, "number of samples per channel"=1000, "error in"=w507) -> ("task out"=w502:refnum<k21>, "data"=w493:waveform(dbl)[], "error out"=w506:errorcluster)  [unwired: 10 in]
        n189 = Enqueue Element(queue=w504, element=w493, error in (no error)=w506) -> (queue out=w503:refnum<queue>, error out=w499:errorcluster)  [unwired: 2 out]
        n190 = Enqueue Element(queue=w500, element=w493, error in (no error)=w499) -> (queue out=w498:refnum<queue>, error out=w497:errorcluster)  [unwired: 2 out]
        n191 = Enqueue Element(queue=w495, element=w493, error in (no error)=w497) -> (queue out=w494:refnum<queue>, error out=w496:errorcluster)  [unwired: 2 out]
      }
    }
    n192 = Unbundle By Name(w393) -> ("code"=w395:i32, "source"=w394:string)
    n193 = call <vilib>:"Simple Error Handler.vi"("error code (no error:0)"=w395, "error source (\" \")"=w394, "type of dialog (OK msg:1)"=w387, "error in (no error)"=w393) -> ("error out"=w388:errorcluster)  [unwired: 1 in, 4 out]
    "Numeric 2" <- w398
    "stop Ind" <- "stop"
  }
  n194 = call <vilib>:"DAQmx Stop Task.vi"("task/channels in"=w28, "error in"=w40) -> ("task out"=w38:refnum<k21>, "error out"=w39:errorcluster)  [unwired: 12 in]
  n195 = call <vilib>:"DAQmx Clear Task.vi"("task in"=w38, "error in"=w39) -> ("error out"=w34:errorcluster)  [unwired: 13 in]
  n196 = Merge Errors(w24, w29, w33, w34, w13) -> (w30:errorcluster)
  n197 = flat-sequence {
    tunnel: w32 -> [w512]
    tunnel: [w512] -> w31
    tunnel: w30 -> [w511]
    tunnel: [w511] -> w18
    tunnel: w20 -> [w509]
    tunnel: [w509] -> w19
    tunnel: [w508] -> w7
    tunnel: w6 -> [w508]
    frame #0 {
      n198 = local write "stop"(FALSE ("create if not found? (T)")) -> ()
    }
  }
  n199 = Release Queue(queue=w19, error in (no error)=w18) -> (error out=w17:errorcluster)  [unwired: 1 in, 2 out]
  n200 = Release Queue(queue=w31, error in (no error)=w17) -> (error out=w9:errorcluster)  [unwired: 1 in, 2 out]
  n201 = Release Queue(queue=w7, error in (no error)=w9) -> (error out=w8:errorcluster)  [unwired: 1 in, 2 out]
  n202 = Unbundle By Name(w8) -> ("code"=w44:i32, "source"=w43:string)
  n203 = call <vilib>:"Simple Error Handler.vi"("error code (no error:0)"=w44, "error source (\" \")"=w43, "error in (no error)"=w8) -> ("error?"=w35:bool, "error out"=w36:errorcluster, "message"=w37:string)  [unwired: 2 in, 2 out]
  n204 = call "Display Message to User"("error in (no error)"=w36, "Enable"=w35, "Message"=w37) -> ()  [unwired: 7 in, 2 out]
